vi "Clear Diagram.vi"(8 "error in (no error)":errorcluster, 11 "Refs In":T1) -> (0 "error out":errorcluster, 3 "Refs":T1)   [LabVIEW 2022 SP3, in "FlexBlocks Support.lvlib"]
uses:
  FlexBlocks Support.lvlib
  SM Refs.ctl
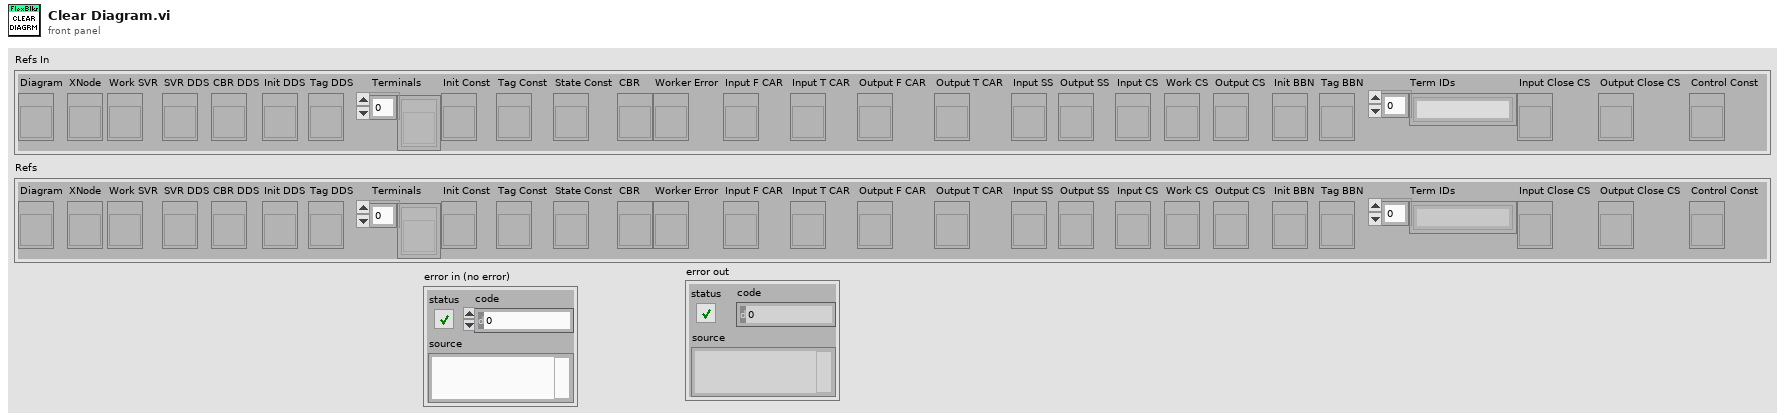
[diagram p1: front panel]
types:
  T1 = typedef "FlexBlocks Support.lvlib/SM Refs.ctl" = cluster{"Diagram":refnum<vi>, "XNode":refnum<vi>, "Work SVR":refnum<vi>, "SVR DDS":refnum<vi>, "CBR DDS":refnum<vi>, "Init DDS":refnum<vi>, "Tag DDS":refnum<vi>, "Terminals":refnum<vi>[], "Init Const":refnum<vi>, "Tag Const":refnum<vi>, "State Const":refnum<vi>, "CBR":refnum<vi>, "Worker Error":refnum<vi>, "Input F CAR":refnum<vi>, "Input T CAR":refnum<vi>, "Output F CAR":refnum<vi>, "Output T CAR":refnum<vi>, "Input SS":refnum<vi>, "Output SS":refnum<vi>, "Input CS":refnum<vi>, "Work CS":refnum<vi>, "Output CS":refnum<vi>, "Init BBN":refnum<vi>, "Tag BBN":refnum<vi>, "Term IDs":string[], "Input Close CS":refnum<vi>, "Output Close CS":refnum<vi>, "Control Const":refnum<vi>}
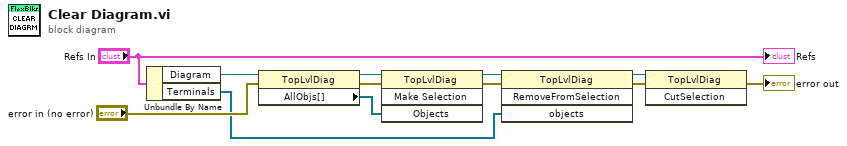
[diagram p0: block diagram]
diagram:
  n1 = Unbundle By Name("Refs In") -> ("Diagram"=w11:refnum<vi>, "Terminals"=w1:refnum<vi>[])
  n2 = property class="TopLvlDiag"(reference=w11, error in="error in (no error)") -> (reference out=w8:refnum<vi>, error out=w6:errorcluster, "AllObjs[]"=w7:refnum<vi>[])
  n3 = invoke class="TopLvlDiag" method="Make Selection"(reference=w8, error in=w6, "Objects"=w7) -> (reference out=w10:refnum<vi>, error out=w9:errorcluster)  [unwired: 1 in, 2 out]
  n4 = invoke class="TopLvlDiag" method="RemoveFromSelection"(reference=w10, error in=w9, "objects"=w1) -> (reference out=w5:refnum<vi>, error out=w4:errorcluster)  [unwired: 1 in, 2 out]
  n5 = invoke class="TopLvlDiag" method="CutSelection"(reference=w5, error in=w4) -> (error out=→"error out":errorcluster)  [unwired: 1 in, 2 out]
  "Refs" <- "Refs In"
